vi "toTimestamp.vi"(7 "Use TAI Offset?":bool, 9 "Fractional Second":dbl format="%#.6f", 10 "Epoch Time (s)":i64, 11 "Epoch (Local)":refnum<class "Epoch.lvclass">) -> (1 "Not a Timestamp?":bool, 2 "Timestamp":timestamp format="%<%H:%M:%S%3u\n%x>T", 3 "Epoch (out)":refnum<class "Epoch.lvclass">)   [LabVIEW 2020, in "Epoch.lvclass"]
uses:
  Epoch.lvclass
  leapSeconds LUT.vi
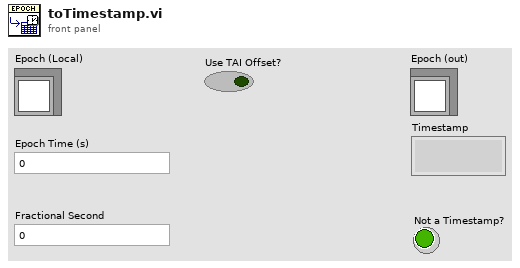
[diagram p1: front panel]
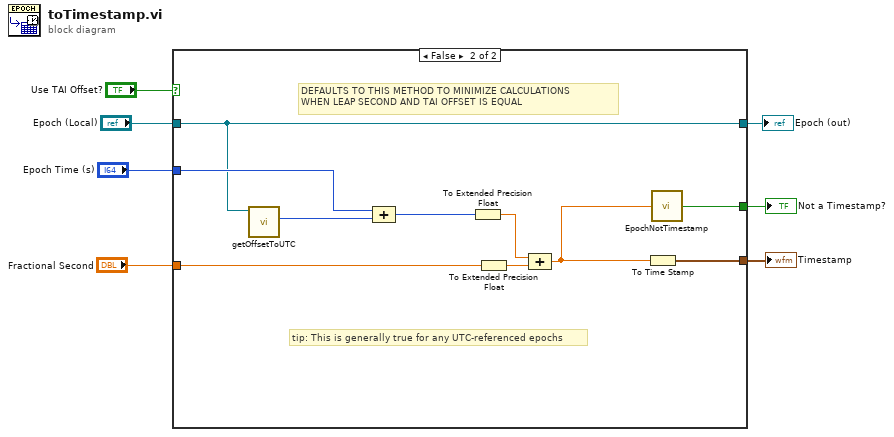
[diagram p0: block diagram]
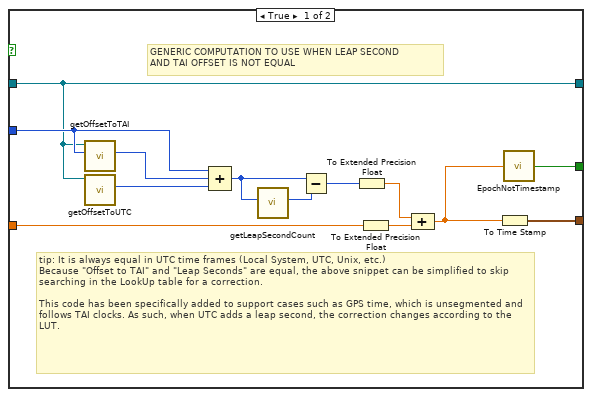
[diagram p2: hidden frame]
diagram:
  n1 = case shown="False" "Use TAI Offset?" {
    tunnel: "Fractional Second" -> [w9 w23]
    tunnel: [w20 w30] -> w6
    tunnel: [w19 w29] -> w1
    tunnel: "Epoch Time (s)" -> [w18 w28]
    tunnel: "Epoch (Local)" -> [w11 w26]
    tunnel: [w11 w26] -> w3
    frame True {
      # "tip: It is always equal in UTC time frames (Local System, UTC, Unix, etc.)\nBecause \"Offset to TAI\" and \"Leap Seconds\" are equal, the above snippet can be simplified to skip searching in the LookUp table for a correction.\n\nThis code has been specifically added to support cases such as GPS time, which is unsegmented and follows TAI clocks. As such, when UTC adds a leap second, the correction changes according to the LUT."
      # "GENERIC COMPUTATION TO USE WHEN LEAP SECOND\nAND TAI OFFSET IS NOT EQUAL"
      n2 = call-dynamic "getOffsetToTAI.vi"("Epoch Time"=w18, "Epoch"=w11) -> ("Offset to TAI"=w16:i64)  [unwired: 9 in]
      n3 = call-dynamic "getOffsetToUTC.vi"("Epoch"=w11) -> ("Offset to UTC"=w12:i64)  [unwired: 10 in]
      n4 = Compound Arithmetic op=ADD(w18, w16, w12) -> (w15:i64)
      n5 = call "getLeapSecondCount.vi"("UTC Epoch Time"=w15) -> ("Leap Seconds"=w14:i64)  [unwired: 10 in]
      n6 = Subtract(x=w15, y=w14) -> (x-y=w13:i64)
      n7 = To Extended Precision Float(1:w13) -> (0:w17:ext)
      n8 = To Extended Precision Float(1:w9) -> (0:w8:ext)
      n9 = Compound Arithmetic op=ADD(w17, w8) -> (w10:ext)
      n10 = To Time Stamp(1:w10) -> (0:w19:timestamp)
      n11 = call "EpochNotTimestamp.vi"("Epoch Time"=w10) -> ("Not a Timestamp?"=w20:bool)  [unwired: 8 in]
    }
    frame False {
      # "tip: This is generally true for any UTC-referenced epochs"
      # "DEFAULTS TO THIS METHOD TO MINIMIZE CALCULATIONS \nWHEN LEAP SECOND AND TAI OFFSET IS EQUAL"
      n12 = call-dynamic "getOffsetToUTC.vi"("Epoch"=w26) -> ("Offset to UTC"=w27:i64)  [unwired: 10 in]
      n13 = Compound Arithmetic op=ADD(w28, w27) -> (w25:i64)
      n14 = To Extended Precision Float(1:w25) -> (0:w24:ext)
      n15 = To Extended Precision Float(1:w23) -> (0:w22:ext)
      n16 = Compound Arithmetic op=ADD(w24, w22) -> (w21:ext)
      n17 = To Time Stamp(1:w21) -> (0:w29:timestamp)
      n18 = call "EpochNotTimestamp.vi"("Epoch Time"=w21) -> ("Not a Timestamp?"=w30:bool)  [unwired: 8 in]
    }
  }
  "Timestamp" <- w1
  "Epoch (out)" <- w3
  "Not a Timestamp?" <- w6
